vi "ocv.vi"(3 "Draw":enum16{"Ewe(t)", "Ece(t)"}(ring), 7 "DLLPath In":path, 8 "error in (no error)":errorcluster, 9 "OCV Parameters":T1={"Rest_time_T"=1.0, "Record_every_dE"=0.01, "Record_every_dT"=0.01, "E_Range"=3, "em"=1, "ce"=0, "tb"=2e-05} {"tb" min=2e-05 max=1 format="%^_3e"; "ce" items=["Standard", "CE to ground"]; "E_Range" items=["±2.5V", "±5V", "±10V", "Auto"]; "Record_every_dT" min=0 format="%.2e"; "Record_every_dE" min=0 max=100 format="%.4f"; "Rest_time_T" min=0 format="%.2f"}, 10 "Channel":u8(ring) items=["1", "2", "3", "4", "5", "6", "7", "8", "9", "10", "11", "12", "13", "14", "15", "16"], 11 "IP adress":string="192.109.209.229") -> (0 "error out":errorcluster, 1 "XY Graph":cluster{"Data 100":dbl[], "Data 100":dbl[]}(graph), 2 "test output":cluster{"Time":dbl[], "Ewet":dbl[], "Ece":dbl[]}, 4 "Exit 2":bool)   [LabVIEW 2022 SP3]
doc: "The Open Circuit Voltage technique consists of a period during which no potantial or current is applied to the working electrode.\nThis VI contain others sub VIs.\nIn general,in this VI, the first thing to do is to start by establishing the connection with the instrument defined by its IP adress, then load the firmware in the channel selected, get the information on the plugged channels, load protocol on a channel, start/stop the protocol, retreive data and draw the graph."
uses:
  Library/EClib Functions/OCVParameters.ctl
  Library/EClib Functions/Parameters.ctl
  Library/EClib Functions/EClib functions.lvlib
panel:
  in  "Display Parameters?":bool caption="Display Parameters"
  out "DllPath":path caption="DLL Path"
  out "LibVersion":string caption="DLL Version"
  in  "Update":bool caption="Start"
  out "Number of points":i32
  out "Data 100":dbl[][](array[numeric]) format="%.2f"
  in  "stop":bool
  in  "Exit":bool
  in  "Start":bool
  # "Instructions:\nBefore running the VI you must type a valid IP adress that corresponds to the instrument.Then press the Run button to execute this VI.\nWhile this VI is running, choose the available channel, enter the OCV parameters or keep the default values, then press the start button to begin the experience. \nThe potential response as a function of the time (Ewe(t), Ece(t)) will be drawn."
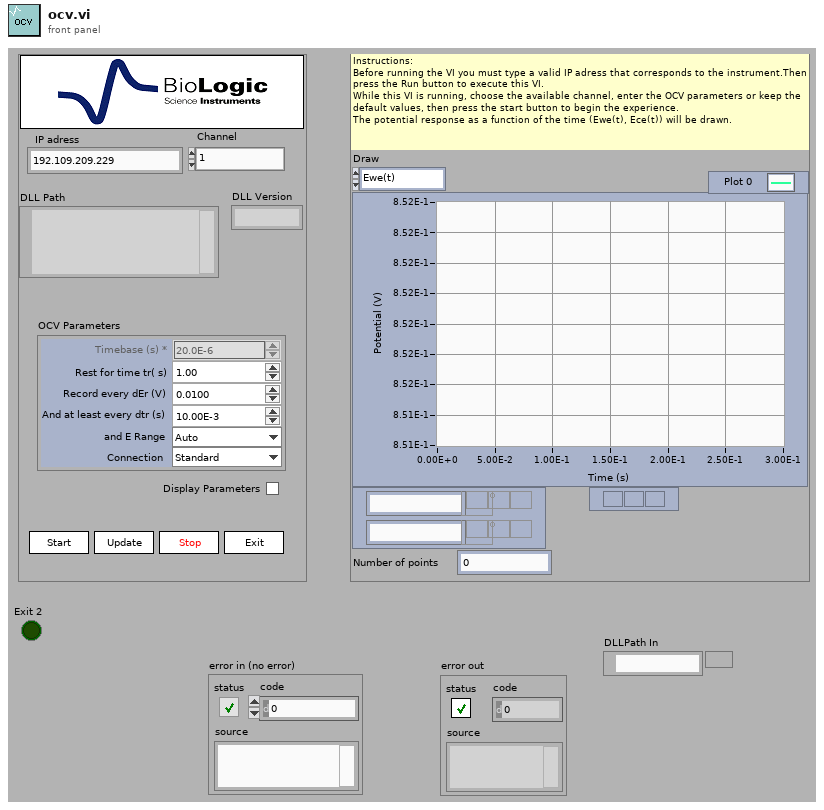
[diagram p1: front panel]
types:
  T1 = typedef "EClib functions.lvlib/OCVParameters.ctl" = cluster{"Rest_time_T":sgl, "Record_every_dE":sgl, "Record_every_dT":sgl, "E_Range":u16, "em":u16, "ce":u16, "tb":sgl}
  T2 = cluster{"LibVersion":string, "StringLength":u32, "DllPath":path}
  T3 = typedef "EClib functions.lvlib/Parameters.ctl" = enum16{"CA", "CASG", "CP", "GEIS", "ISCAN", "OCV", "PEIS", "SCCX", "SGEIS", "SPEIS", "VSCAN", "MP"}
  T4 = typedef "EClib functions.lvlib/TechniqueParameters.ctl" = cluster{"String Label":string, "Type":i32, "Valeur":i32, "Index":i32}
  T5 = cluster{"string before end tag":string, i32, i32, i32}[]
  T6 = cluster{"IRQskipped":i32, "NbRaws":i32, "NbCols":i32, "Technique Index":i32, "TechniqueID":i32, "PrcessIndex":i32, "loop":i32, "StartTime":dbl, "MuxPad":i32}
  T7 = cluster{"State":i32, "MemFilled":i32, "TimeBase":sgl, " Ewe":sgl, " EweRangeMin":sgl, " EweRangeMax":sgl, "Ece":sgl, "EceRangeMin":sgl, "EceRangeMax":sgl, "Eoverflow":i32, "I":sgl, "IRange":i32, "Ioverflow":i32, "ElapsedTime":sgl, "Freq":sgl, "Rcomp":sgl, "Saturation":sgl, "OptErr":i32, "OptPos":i32}
  T8 = cluster{"Label":string, "type":i32, "valeur":u32, "index":i32}[]
  T9 = cluster{"Data 100":dbl[], "Data 100":dbl[], "Data 100":dbl[]}
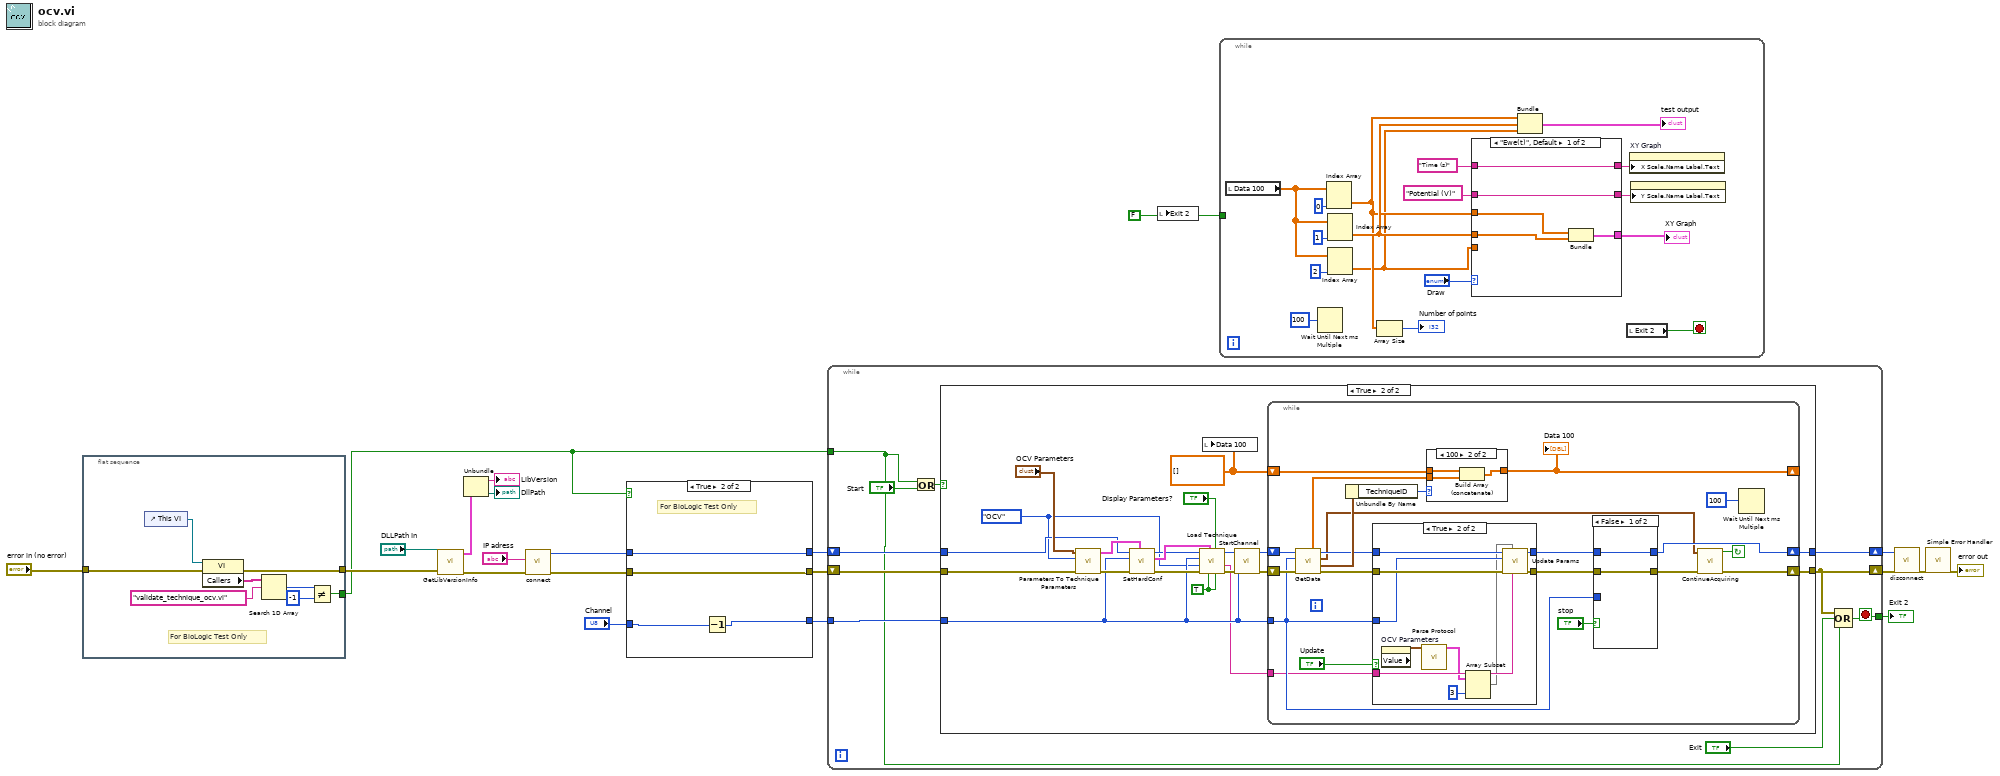
[diagram p0: block diagram]
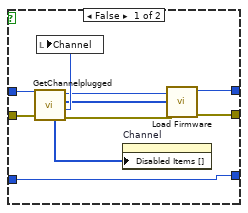
[diagram p2: hidden frame]
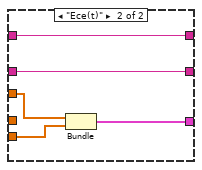
[diagram p3: hidden frame]
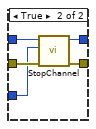
[diagram p6: hidden frame]
diagram:
  w20 = FALSE ("Exit 2")
  n1 = flat-sequence {
    tunnel: "error in (no error)" -> [w28]
    tunnel: [w27] -> w5
    tunnel: [w22] -> w3
    frame #0 {
      # "For BioLogic Test Only"
      n2 = control-ref of="This VI"() -> (w29:refnum<vi>)
      n3 = property class="VI"(reference=w29, error in=w28) -> (error out=w27:errorcluster, "Callers"=w26:string[])  [unwired: 1 out]
      n4 = Search 1D Array(1D array=w26, element="validate_technique_ocv.vi") -> (index of element=w24:i32)  [unwired: 1 in]
      n5 = Not Equal?(x=w24, y=-1) -> (x != y?=w22:bool)
    }
  }
  n6 = call "GetLibVersionInfo.vi"("error in (no error)"=w5, "DLLPath"="DLLPath In") -> ("error out"=w10:errorcluster, "LibInfo"=w13:T2)  [unwired: 8 in]
  n7 = Unbundle(w13) -> ("LibVersion"=→"LibVersion":string, "DllPath"=→"DllPath":path)  [unwired: 1 out]
  n8 = call "connect.vi"("error in (no error)"=w10, "IP"="IP adress") -> ("error out"=w9:errorcluster, "ID Out"=w8:i32)  [unwired: 5 in, 3 out]
  n9 = case shown="True" w3 {
    tunnel: [w39 w43] -> w17
    tunnel: [w38 w42] -> w16
    tunnel: w9 -> [w36 w42]
    tunnel: w8 -> [w35 w43]
    tunnel: "Channel" -> [w30 w41]
    tunnel: [w30 w40] -> w6
    frame False {
      n10 = call "GetChannelplugged.vi"("error in (no error)"=w36, "ID In"=w35) -> ("error out"=w34:errorcluster, "FirstPluggedChannel"=w37:u8, "PluggedChannels"=w33:u8[], "ID Out"=w32:i32, "DisabledChannels"=w31:i32[])  [unwired: 5 in]
      n11 = local write "Channel"(w37) -> ()
      n12 = property on="Channel" class="Ring (strict)"("Disabled Items []"=w31) -> ()  [unwired: 2 in, 2 out]
      n13 = call "Load Firmware.vi"("error in (no error)"=w34, "Channels"=w33, "ID In"=w32) -> ("error out"=w38:errorcluster, "ID Out"=w39:i32)  [unwired: 6 in, 1 out]
    }
    frame True {
      # "For BioLogic Test Only"
      n14 = Decrement(x=w41) -> (x-1=w40:u8)
    }
  }
  n15 = while {
    shift-right: [w49] -> w15
    shift-left: w16 -> [w52]
    tunnel: [w48] -> w21
    shift-right: [w53] -> w18
    shift-left: w17 -> [w51]
    tunnel: w6 -> [w47]
    tunnel: w3 -> [w44]
    stop <- w48 stop-if-true
    n16 = Or(x=w44, y="Start") -> (x .or. y?=w45:bool)
    n17 = case shown="True" w45 {
      tunnel: w47 -> [_ w59]
      tunnel: [w55 w75] -> w49
      tunnel: w52 -> [w55 w60]
      tunnel: w51 -> [w54 w58]
      tunnel: [w54 w73] -> w53
      frame False {
      }
      frame True {
        w57 = Parameters."OCV" ("Parameters")
        w71 = TRUE ("First Protocol")
        w74 = dbl[][] []
        n18 = call "Parameters To Technique Parameters.vi"("error in (no error)"=w60, "Parameters"=w57, "ParameterIN"="OCV Parameters") -> ("error out"=w62:errorcluster, "Params Values"=w63:T4[])  [unwired: 7 in]
        n19 = call "SetHardConf.vi"("Params Values"=w63, "error in (no error)"=w62, "Channel"=w59, "ID In"=w58) -> ("error out"=w64:errorcluster, "Params Values Trimed"=w66:T5, "ID Out"=w65:i32)  [unwired: 5 in]
        n20 = call "Load Technique.vi"("Last Protocol"=w71, "Display Parameters?"="Display Parameters?", "First Protocol"=w71, "TechniqueParameters"=w66, "error in (no error)"=w64, "Parameters"=w57, "Selected Channel"=w59, "ID In"=w65) -> ("error out"=w67:errorcluster, "Fichier .ecc"=w56:string, "ID  Out"=w69:i32)  [unwired: 1 in]
        n21 = local write "Data 100"(w74) -> ()
        n22 = call "StartChannel.vi"("error in (no error)"=w67, "Channel"=w59, "ID In"=w69) -> ("error out"=w70:errorcluster, "ID Out"=w68:i32)  [unwired: 7 in]
        n23 = while {
          shift-right: [w80] -> w75
          shift-left: w70 -> [w96]
          shift-right: [w94] -> _
          shift-left: w74 -> [w93]
          tunnel: w59 -> [w86]
          shift-right: [w81] -> w73
          shift-left: w68 -> [w84]
          tunnel: w56 -> [w76]
          stop <- w77 continue-if-true
          n24 = call "GetData.vi"("error in (no error)"=w96, "Channel"=w86, "ID In"=w84) -> ("error out"=w88:errorcluster, "Data information"=w90:T6, "Current values"=w78:T7, "ID Out"=w82:i32, "Data"=w85:dbl[][])  [unwired: 1 in, 3 out]
          n25 = Unbundle By Name(w90) -> ("TechniqueID"=w91:i32)
          n26 = case shown="True" "Update" {
            tunnel: w88 -> [w98 w108]
            tunnel: [w98 w107] -> w87
            tunnel: w82 -> [w97 w106]
            tunnel: w86 -> [_ w105]
            tunnel: w76 -> [_ w104]
            tunnel: [w97 w101] -> w83
            frame False {
            }
            frame True {
              n27 = property on="OCV Parameters" class="Clust (strict)"() -> ("Value"=w100:T1)  [unwired: 2 in, 2 out]
              n28 = call "Parse Protocol.vi"("Protocol Cluster"=w100) -> ("Params Values"=w99:T8)  [unwired: 9 in, 1 out]
              n29 = Array Subset(array=w99, length=3) -> (w102:T8)  [unwired: 1 in]
              n30 = call "Update Params.vi"("EccFileName"=w104, "Params"=w102, "error in (no error)"=w108, "Channel"=w105, "ID"=w106) -> ("error out"=w107:errorcluster, "ID Out"=w101:i32)  [unwired: 5 in]
            }
          }
          n31 = case shown="100" w91 {
            tunnel: w85 -> [_ w119]
            tunnel: [w116 w118] -> w94
            tunnel: w93 -> [w116 w117]
            frame 0, Default {
            }
            frame 100 {
              n32 = Build Array (concatenate)(w117, w119) -> (w118:dbl[][])
            }
          }
          "Data 100" <- w94
          n33 = case shown="False" "stop" {
            tunnel: [w110 w115] -> w79
            tunnel: w87 -> [w110 w114]
            tunnel: w86 -> [_ w113]
            tunnel: w83 -> [w109 w112]
            tunnel: [w109 w111] -> w81
            frame False {
            }
            frame True {
              n34 = call "StopChannel.vi"("error in (no error)"=w114, "Channel"=w113, "ID In"=w112) -> ("error out"=w115:errorcluster, "ID Out"=w111:i32)  [unwired: 7 in]
            }
          }
          n35 = call "ContinueAcquiring.vi"("error in"=w79, "Current values"=w78) -> ("error out"=w80:errorcluster, "ContinueAcquiring?"=w77:bool)  [unwired: 8 in]
          n36 = Wait Until Next ms Multiple(millisecond multiple=u32 100) -> ()  [unwired: 1 out]
        }
      }
    }
    n37 = Compound Arithmetic op=OR(w49, "Exit", w44) -> (w48:bool)
  }
  "Exit 2" <- w21
  n38 = local write "Exit 2"(w20) -> ()
  n39 = while {
    tunnel: w20 -> [_]
    stop <- w133 stop-if-true
    n40 = local read "Data 100"() -> (w131:dbl[][])
    n41 = Wait Until Next ms Multiple(millisecond multiple=u32 100) -> ()  [unwired: 1 out]
    n42 = Index Array(array=w131, index (col)=0 ("Index")) -> (element=w124:dbl[])  [unwired: 1 in]
    n43 = Index Array(array=w131, index (col)=1 ("Index")) -> (element=w125:dbl[])  [unwired: 1 in]
    n44 = Index Array(array=w131, index (col)=2 ("indice désactivé (col)")) -> (element=w123:dbl[])  [unwired: 1 in]
    n45 = Array Size(array=w124) -> (size(s)=→"Number of points":i32)
    n46 = case shown="\"Ewe(t)\", Default" "Draw" {
      tunnel: "Time (s)" ("Y Scale.Name Label.Text") -> [w141 w146]
      tunnel: [w141 w146] -> w128
      tunnel: "Potential (V)" ("Y Scale.Name Label.Text") -> [w140 w145]
      tunnel: [w140 w145] -> w126
      tunnel: w124 -> [w138 w142]
      tunnel: w125 -> [w137 _]
      tunnel: w123 -> [_ w144]
      tunnel: [w139 w143] -> w121
      frame "Ewe(t)", Default {
        n47 = Bundle("Data 100"=w138, "Data 100"=w137) -> (w139:cluster{"Data 100":dbl[], "Data 100":dbl[]})  [unwired: 1 in]
      }
      frame "Ece(t)" {
        n48 = Bundle("Data 100"=w142, "Data 100"=w144) -> (w143:cluster{"Data 100":dbl[], "Data 100":dbl[]})  [unwired: 1 in]
      }
    }
    "XY Graph" <- w121
    n49 = Bundle("Data 100"=w124, "Data 100"=w125, "Data 100"=w123) -> (→"test output":T9)  [unwired: 1 in]
    n50 = local read "Exit 2"() -> (w133:bool)
    n51 = property on="XY Graph" class="XYGraph (strict)"("X Scale.Name Label.Text"=w128) -> ()  [unwired: 2 in, 2 out]
    n52 = property on="XY Graph" class="XYGraph (strict)"("Y Scale.Name Label.Text"=w126) -> ()  [unwired: 2 in, 2 out]
  }
  n53 = call "disconnect.vi"("error in (no error)"=w15, "ID In"=w18) -> ("error out"=w14:errorcluster)  [unwired: 9 in]
  n54 = call <vilib>:"Simple Error Handler.vi"("error in (no error)"=w14) -> ("error out"=→"error out":errorcluster)  [unwired: 4 in, 4 out]
